vi "Camera Configure.vi"(8 "error in":errorcluster) -> (0 "error out":errorcluster)   [LabVIEW 2012]
doc: "The Grab and Attributes Setup example VI allows the user to view the current attributes and settings, update attribute settings, acquire images continuously, and display the images in an image control."
uses:
  <vilib>/userdefined/High Color/IMAQdx.ctl
  Process Controller 3.0/Control code/Camera/Camera source code/Interface Inputs.ctl
  Process Controller 3.0/Control code/Camera/Camera source code/Rotate.ctl
  Process Controller 3.0/Control code/Camera/Camera source code/Image File Type.ctl
  <vilib>/vision/driver/IMAQdx.llb/IMAQdx Acquisition Mode.ctl
  <vilib>/vision/driver/IMAQdx.llb/IMAQdx Buffer Number Mode.ctl
  DAC project/Calibration and Function folders.ctl
  <vilib>/vision/driver/NI_Vision_Acquisition_Software.lvlib
  Process Controller 3.0/Control code/Camera/Camera SubVIs.lvlib
panel:
  out "Global Rectangle":i32[](array[numeric])
  in  "Grab":bool
  in  "Cancel":bool
  in  "OK":bool
  in  "Tab Contro Mainl":T1(tab)
  in  "Attribute Tree":string(tree)
  in  "Camera Name":T2
  in  "Tab Control":T3(tab)
  in  "U32 Value Control":u32(slide) min=480 max=6291456 step=1 scale=5662310.4..6291456.0
  in  "DBL Value Control":dbl(slide) min=0.0 max=3.999 step=1.0 scale=0.0..3.999
  in  "String Value Control":string
  in  "Enum Value Control":u32(ring) items=["160x120 MJPG 30.00fps", "160x120 YUY2 30.00fps", "176x144 MJPG 30.00fps", "176x144 YUY2 30.00fps", "320x240 MJPG 30.00fps", "320x240 YUY2 30.00fps", "352x288 MJPG 30.00fps", "352x288 YUY2 30.00fps", "640x480 MJPG 30.00fps", "640x480 YUY2 30.00fps", "1024x768 MJPG 30.00fps", "1024x768 YUY2 12.00fps", "1280x720 MJPG 15.00fps", "1280x720 YUY2 10.00fps", "1280x1024 MJPG 15.00fps", "1280x1024 YUY2 7.50fps", "1600x1200 MJPG 15.00fps", "1600x1200 YUY2 5.00fps", "1920x1080 MJPG 15.00fps", "1920x1080 YUY2 4.00fps", "2048x1536 MJPG 15.00fps", "2048x1536 YUY2 3.00fps"]
  in  "Boolean Value Control":bool=TRUE
  in  "Command Value Control":bool
  out "Units":string
  out "Tooltip":string
  out "Image":T4(plugin-control)
  in  "Interface inputs":T5={"Elevation of top of Field of View (cm)"=10.0, "Field of View Height (cm)"=-0.1, "Smooth Length (cm)"=5.0, "Min derivative magnitude"=5.0, "Color Plane"=enum."Green"} {"Smooth Length (cm)" min=0.01 max=1000.0 step=0.1; "Field of View Height (cm)" min=0.1 max=1000.0 step=0.1}
  in  "File Type":T6
  in  "Image Save Rate (s)":dbl=5.0 min=0.05 step=0.05 format="%#_3f"
  in  "Image folder":path
  in  "Record images":bool
  in  "Rotate Image":T7
  out "Buffer Number":u32
  out "Interface elevation":dbl format="%#_3g"
  out "derivative magnitude":dbl format="%#_3g"
  out "Tab Control Ref":T8
  # "These settings are saved in the  ProCoDA configuration file. The Region of Interest is also saved in the configuration file."
  # "Turn of the camera external code in Process Controller prior to using this software. Only one application can interface with the camera at a time. After the camera is configured you can close this application and open the camera external code in Process Controller.\n\nConfigure the camera (light settings, resolution etc.) and then test those settings by acquiring images. \n \nUse the rectangle tool in the image to define the region of interest where the floc water interface will appear.\nThe region of interest is saved in a configuration file.\n\nChoose a folder to save images during the experiment.\nChoose the rate at which images are saved.\n\nUse TIFF files if you plan to do pixel by pixel image analysis and thus don't want image compression. Otherwise JPEG is a good option to reduce file size. \n\nWhen testing to see if the interface is correctly identified, a horizontal black line with a height equal to the smoothing length will appear on the image when an interface is found. If an interface is found, but the line does not appear that is due to the fact the image is reduced in size and the pixels containing the line are not being displayed. You can zoom on the image to see the line."
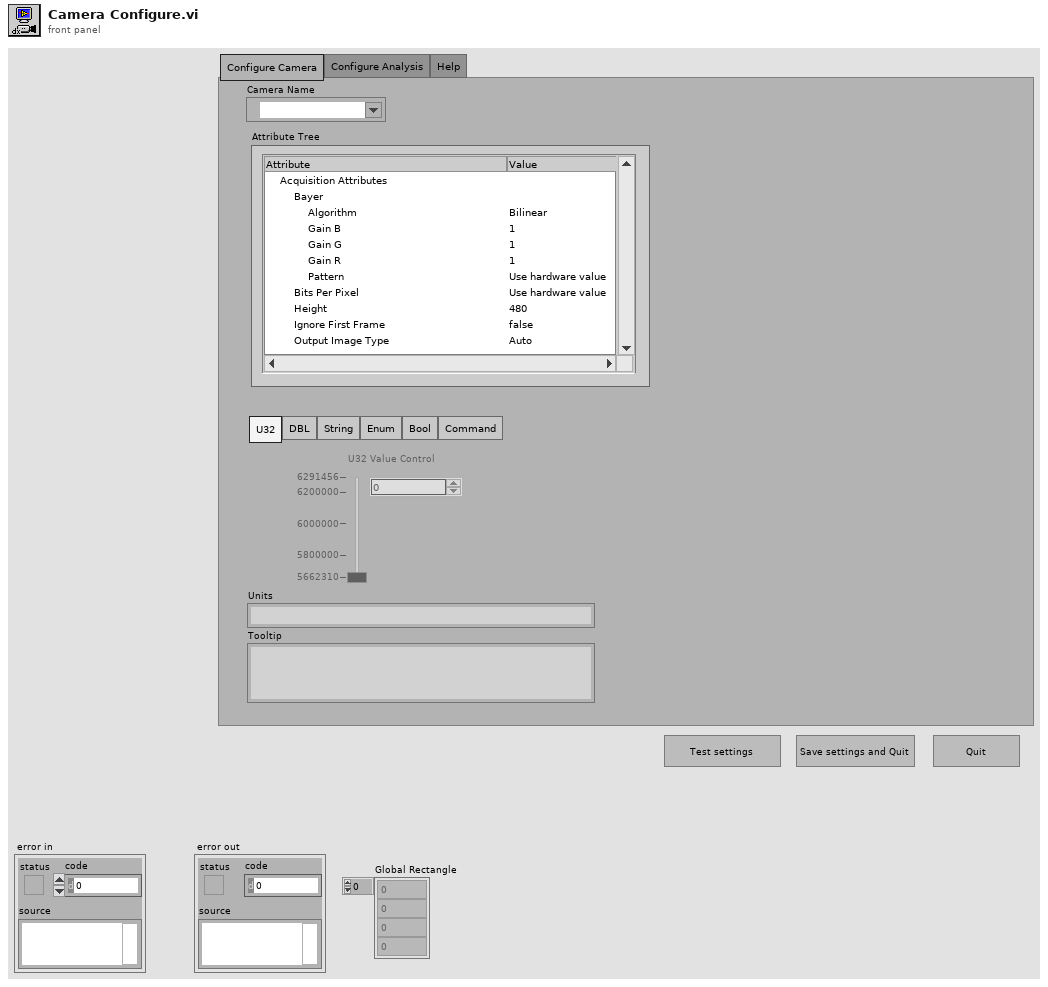
[diagram p1: front panel]
types:
  T1 = enum32{"Configure Camera", "Configure Analysis", "Help"}
  T2 = typedef "IMAQdx.ctl" = refnum<k21>
  T3 = enum32{"U32", "DBL", "String", "Enum", "Bool", "Command"}
  T4 = typedef "IMAQ Image.ctl" = refnum<image>
  T5 = typedef "Camera SubVIs.lvlib/Interface Inputs.ctl" = cluster{"Elevation of top of Field of View (cm)":dbl, "Field of View Height (cm)":dbl, "Smooth Length (cm)":dbl, "Min derivative magnitude":dbl, "Color Plane":enum16{"Red", "Green", "Blue", "Combined"}}
  T6 = typedef "Camera SubVIs.lvlib/Image File Type.ctl" = enum16{"BMP", "JPEG", "JPEG 2000", "PNG", "PNG with Vision Info", "TIFF"}
  T7 = typedef "Camera SubVIs.lvlib/Rotate.ctl" = enum16{"None", "CW", "CCW"}
  T8 = cluster{"Tab Control":refnum<vi>, "U32 Value Control":refnum<vi>, "DBL Value Control":refnum<vi>, "String Value Control":refnum<vi>, "Enum Value Control":refnum<vi>, "Boolean Value Control":refnum<vi>, "Command Value Control":refnum<vi>}
  T9 = enum32{"invalid app kind", "Development System", "Run Time System", "Student Edition", "Embedded LabVIEW", "Evaluation", "Custom"}
  T10 = cluster{"Global Rectangle":i32[], "Contours":cluster{"Contour Type":u32, "ROI Type":u32, "Points":i32[]}[]}
  T11 = typedef "NI_Vision_Acquisition_Software.lvlib/IMAQdx Acquisition Mode.ctl" = enum32{"One Shot", "Continuous"}
  T12 = enum8{"Enabled", "Disabled", "Disabled and Grayed Out"}
  T13 = typedef "Calibration and Function folders.ctl" = enum16{"Sensors", "Functions", "Config File", "UserAppFolder"}
  T14 = typedef "Image Type" = u32
  T15 = typedef "NI_Vision_Acquisition_Software.lvlib/IMAQdx Buffer Number Mode.ctl" = enum32{"Next", "Last", "Buffer Number"}
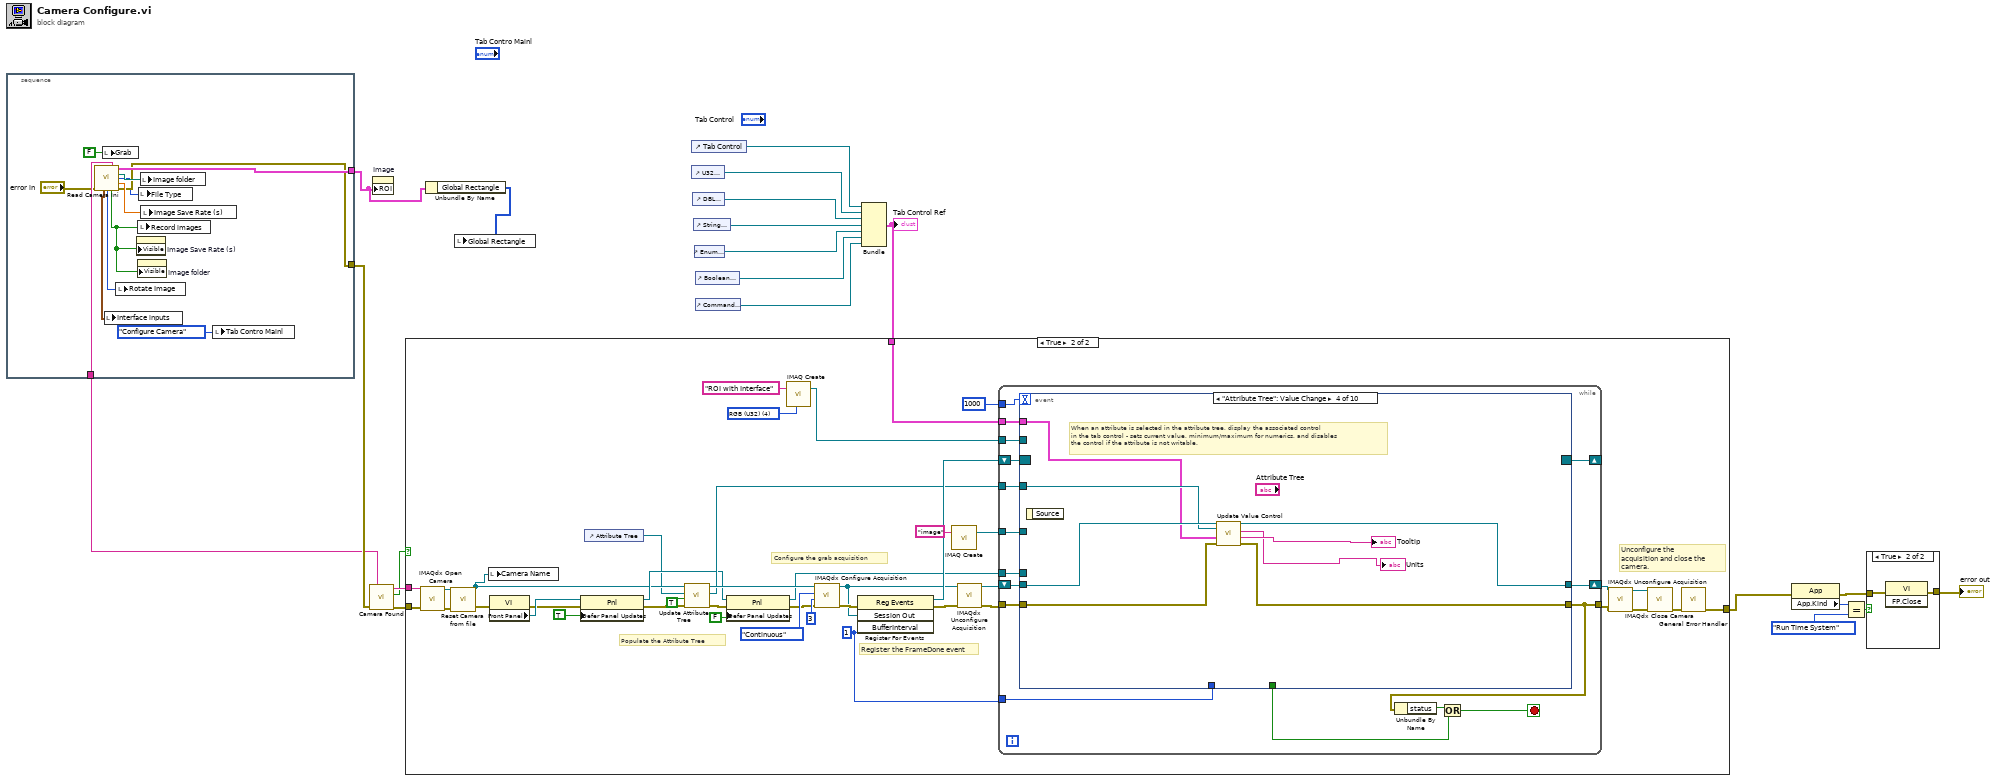
[diagram p0: block diagram]
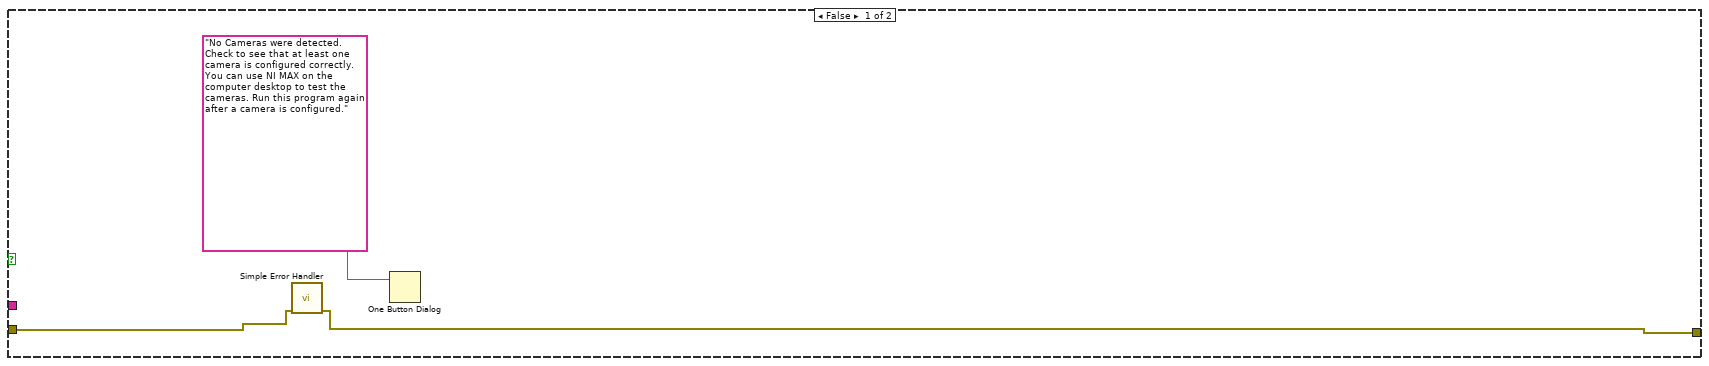
[diagram p3: hidden frame]
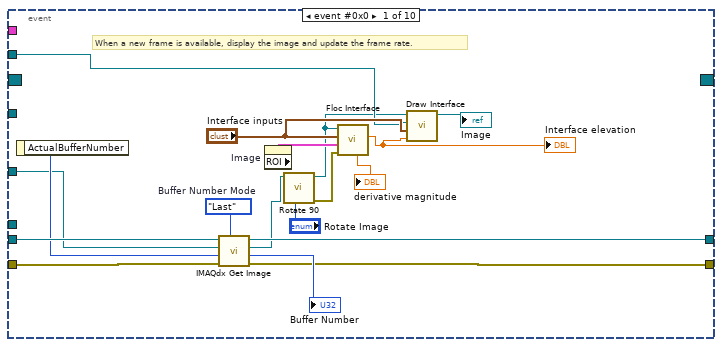
[diagram p4: hidden frame]
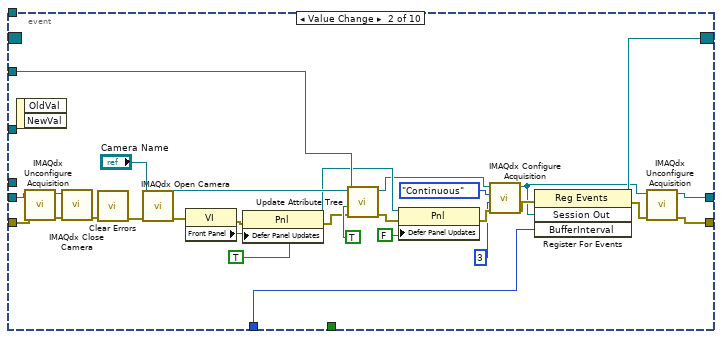
[diagram p5: hidden frame]
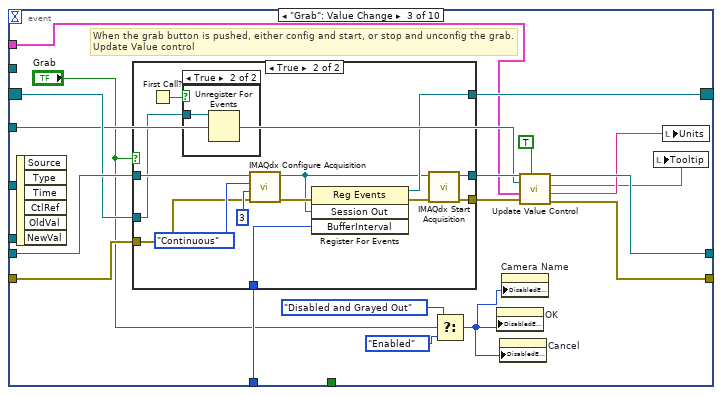
[diagram p6: hidden frame]
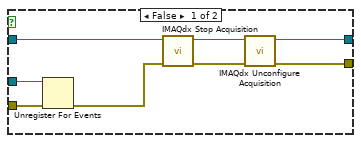
[diagram p7: hidden frame]
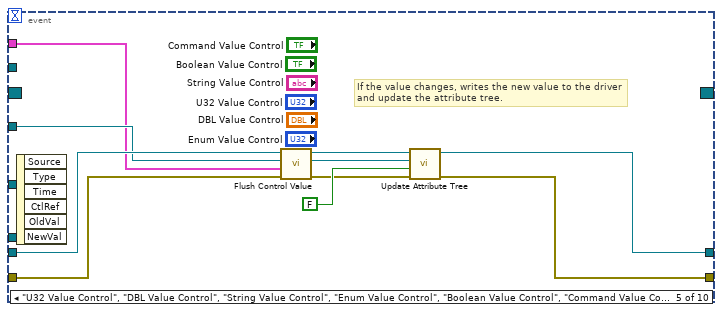
[diagram p9: hidden frame]
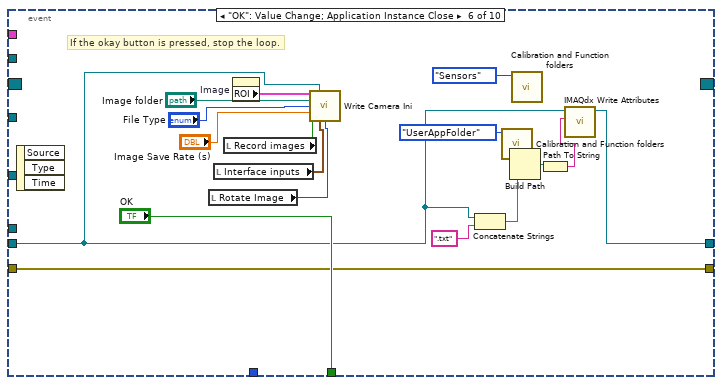
[diagram p10: hidden frame]
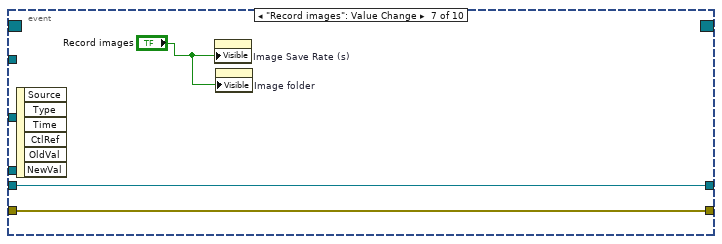
[diagram p11: hidden frame]
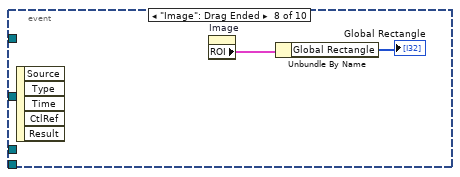
[diagram p12: hidden frame]
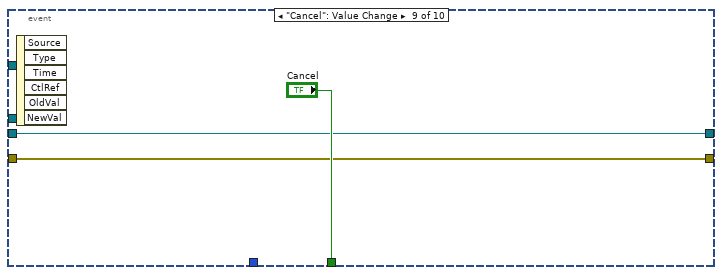
[diagram p13: hidden frame]
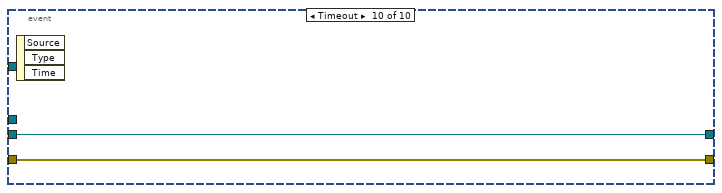
[diagram p14: hidden frame]
diagram:
  n1 = stacked-sequence {
    tunnel: [w33] -> w14
    tunnel: [w24] -> w12
    tunnel: [w26] -> w11
    frame #0 {
      n2 = call "Read Camera Ini.vi"("error in (no error)"="error in") -> ("CameraName"=w26:string, "ROI"=w33:T10, "Image folder"=w31:path, "File Type"=w22:T6, "Image Save Rate (s)"=w30:dbl, "Interface inputs"=w27:T5, "Rotate"=w23:T7, "Record images"=w29:bool, "error out"=w24:errorcluster)  [unwired: 6 in]
      n3 = local write "Grab"(FALSE ("Grab")) -> ()
      n4 = local write "Interface inputs"(w27) -> ()
      n5 = local write "Rotate Image"(w23) -> ()
      n6 = property on="Image Save Rate (s)" class="DigNum (strict)"("Visible"=w29) -> ()  [unwired: 2 in, 2 out]
      n7 = local write "Record images"(w29) -> ()
      n8 = property on="Image folder" class="Path"("Visible"=w29) -> ()  [unwired: 2 in, 2 out]
      n9 = local write "File Type"(w22) -> ()
      n10 = local write "Image folder"(w31) -> ()
      n11 = local write "Image Save Rate (s)"(w30) -> ()
      n12 = local write "Tab Contro Mainl"(T1."Configure Camera" ("Tab Contro Mainl")) -> ()
    }
  }
  n13 = call "Camera Found.vi"("error in"=w12, "CameraName"=w11) -> ("error out"=w9:errorcluster, "Camera Found"=w8:bool, "CameraName out"=w10:string)  [unwired: 7 in]
  n14 = property on="Image" class="ImageControl"("ROI"=w14) -> ()  [unwired: 2 in, 2 out]
  n15 = Unbundle By Name(w14) -> ("Global Rectangle"=w13:i32[])
  n16 = local write "Global Rectangle"(w13) -> ()
  n17 = control-ref of="Tab Control"() -> (w21:refnum<vi>)
  n18 = control-ref of="U32 Value Control"() -> (w19:refnum<vi>)
  n19 = control-ref of="DBL Value Control"() -> (w18:refnum<vi>)
  n20 = control-ref of="String Value Control"() -> (w20:refnum<vi>)
  n21 = control-ref of="Enum Value Control"() -> (w17:refnum<vi>)
  n22 = control-ref of="Boolean Value Control"() -> (w16:refnum<vi>)
  n23 = control-ref of="Command Value Control"() -> (w15:refnum<vi>)
  n24 = Bundle("Tab Control"=w21, "U32 Value Control"=w19, "DBL Value Control"=w18, "String Value Control"=w20, "Enum Value Control"=w17, "Boolean Value Control"=w16, "Command Value Control"=w15) -> (w1:T8)  [unwired: 1 out]
  "Tab Control Ref" <- w1
  n25 = case shown="True" w8 {
    tunnel: [w34 w54] -> w3
    tunnel: w10 -> [_ w44]
    tunnel: w9 -> [w36 w43]
    tunnel: w1 -> [_ w38]
    frame False {
      n26 = call <vilib>:"Simple Error Handler.vi"("error in (no error)"=w36) -> ("error out"=w34:errorcluster)  [unwired: 4 in, 4 out]
      n27 = One Button Dialog(message="No Cameras were detected. Check to see that at least one camera is configured correctly. You can use NI MAX on the computer desktop to test the cameras. Run this program again after a camera is configured.") -> ()  [unwired: 1 in, 1 out]
    }
    frame True {
      w50 = T14 4 items=["Grayscale (U8)", "Grayscale (I16)", "Grayscale (SGL)", "Complex (CSG)", "RGB (U32)", "HSL (U32)", "RGB (U64)", "Grayscale (U16)"] ("Image Type")
      w60 = u32 1 ("BufferInterval")
      # "Unconfigure the acquisition and close the camera."
      # "Register the FrameDone event"
      # "Configure the grab acquisition"
      # "Populate the Attribute Tree"
      n28 = call <vilib>:"IMAQdx Open Camera.vi"("error in"=w43, "Session In"=w44) -> ("error out"=w48:errorcluster, "Session Out"=w47:T2)  [unwired: 1 in, 7 out]
      n29 = call "Reset Camera from file.vi"("error in"=w48, "Refnum in"=w47) -> ("error out"=w46:errorcluster, "Refnum out"=w42:T2)  [unwired: 8 in]
      n30 = local write "Camera Name"(w42) -> ()
      n31 = property class="VI"(error in=w46) -> (error out=w61:errorcluster, "Front Panel"=w62:refnum<vi>)  [unwired: 1 in, 1 out]
      n32 = property class="Pnl"(reference=w62, error in=w61, "Defer Panel Updates"=TRUE) -> (reference out=w65:refnum<vi>, error out=w69:errorcluster)
      n33 = control-ref of="Attribute Tree"() -> (w37:refnum<vi>)
      n34 = call "Update Attribute Tree.vi"("error in"=w69, "Flush Tree?"=TRUE, "Tree Control In"=w37, "Camera Name In"=w42) -> ("error out"=w68:errorcluster, "Tree Control Out"=w70:refnum<vi>, "Session Out"=w72:T2)  [unwired: 5 in]
      n35 = property class="Pnl"(reference=w65, error in=w68, "Defer Panel Updates"=FALSE) -> (reference out=w64:refnum<vi>, error out=w66:errorcluster)
      n36 = call "IMAQ Create"("Image Name"="ROI with Interface", "Image Type"=w50) -> ("New Image"=w49:T4)  [unwired: 3 in, 1 out]
      n37 = call <vilib>:"IMAQdx Configure Acquisition.vi"("error in"=w66, "Number of Buffers"=u32 3, "Continuous?"=IMAQdx_Acquisition_Mode."Continuous", "Session In"=w72) -> ("error out"=w75:errorcluster, "Session Out"=w57:T2)  [unwired: 6 out]
      n38 = register-events(error in=w75, w57, w60) -> (reference out=w74:refnum<event-registration>, error out=w59:errorcluster)  [unwired: 1 in]
      n39 = call "IMAQ Create"("Image Name"="image") -> ("New Image"=w52:T4)  [unwired: 3 in, 2 out]
      n40 = call <vilib>:"IMAQdx Unconfigure Acquisition.vi"("error in"=w59, "Session In"=w57) -> ("error out"=w58:errorcluster, "Session Out"=w56:T2)  [unwired: 8 out]
      n41 = while {
        tunnel: w58 -> [w90]
        tunnel: [w88] -> w55
        tunnel: w52 -> [w89]
        tunnel: 1000 -> [w86]
        tunnel: w70 -> [w85]
        tunnel: w64 -> [w84]
        tunnel: w60 -> [w82]
        shift-right: [w81] -> _
        shift-left: w74 -> [w87]
        shift-right: [w80] -> w53
        shift-left: w56 -> [w91]
        tunnel: w49 -> [w79]
        tunnel: w38 -> [w78]
        stop <- w93 stop-if-true
        n42 = event shown="[3] \"Attribute Tree\": Value Change" {
          selector: w87 -> [_ _ w155 _ _ _ _ _ _ _]
          dyn-events: [_ w118 w157 _ _ _ _ _ _ _] -> w81
          timeout: w86 -> [_ _ _ _ _ _ _ _ _ _]
          tunnel: w91 -> [w111 w139 w158 w188 w197 w205 w218 _ w223 w225]
          tunnel: w90 -> [w110 w138 w154 w186 w198 w215 w217 _ w222 w226]
          tunnel: w89 -> [w103 _ _ _ _ _ _ _ _ _]
          tunnel: [w104 w114 w152 w187 w192 w210 w218 _ w223 w225] -> w80
          tunnel: [w99 w116 w150 w185 w189 w215 w217 _ w222 w226] -> w88
          tunnel: w85 -> [_ w136 w149 w184 w195 _ _ _ _ _]
          tunnel: w84 -> [_ _ _ _ _ _ _ _ _ _]
          tunnel: [_ _ _ _ _ "OK" _ _ "Cancel" _] -> w83
          tunnel: w82 -> [_ w119 w156 _ _ _ _ _ _ _]
          tunnel: w79 -> [w100 _ _ _ _ _ _ _ _ _]
          tunnel: w78 -> [_ _ w141 w183 w191 _ _ _ _ _]
          event event #0x0 {
            w109 = IMAQdx_Buffer_Number_Mode."Last"  # Buffer Number Mode
            # "When a new frame is available, display the image and update the frame rate."
            n43 = event-data() -> ("ActualBufferNumber"=w108:u32)  [unwired: 1 out]
            n44 = call <vilib>:"IMAQdx Get Image.vi"("Buffer Number Mode (Next)"=w109, "error in"=w110, "Buffer Number In"=w108, "Image In"=w103, "Session In"=w111) -> ("error out"=w99:errorcluster, "Buffer Number Out"=→"Buffer Number":u32, "Image Out"=w97:T4, "Session Out"=w104:T2)  [unwired: 3 out]
            n45 = property on="Image" class="ImageControl"() -> ("ROI"=w106:T10)  [unwired: 2 in, 2 out]
            n46 = call "Rotate 90.vi"("Rotate"="Rotate Image", "Image Src"=w97) -> ("error out"=w94:errorcluster, "Image Dst Out"=w96:T4)  [unwired: 8 in]
            n47 = call "Floc Interface.vi"("error in"=w94, "ROI"=w106, "Interface inputs"="Interface inputs", "Image"=w96) -> ("Interface elevation"=w102:dbl, "min value"=→"derivative magnitude":dbl)  [unwired: 4 in, 2 out]
            "Interface elevation" <- w102
            n48 = call "Draw Interface.vi"("Interface elevation"=w102, "Interface inputs"="Interface inputs", "Image Dst"=w100, "Image"=w96) -> ("Image out"=→"Image":T4)  [unwired: 7 in]
          }
          event Value Change {
            n49 = event-data() -> ()  [unwired: 3 out]
            n50 = call <vilib>:"IMAQdx Unconfigure Acquisition.vi"("error in"=w138, "Session In"=w139) -> ("error out"=w140:errorcluster, "Session Out"=w137:T2)  [unwired: 8 out]
            n51 = call <vilib>:"IMAQdx Close Camera.vi"("error in"=w140, "Session In"=w137) -> ("error out"=w133:errorcluster)  [unwired: 9 out]
            n52 = call <vilib>:"Clear Errors.vi"("error in (no error)"=w133) -> ("error out"=w132:errorcluster)  [unwired: 6 in]
            n53 = call <vilib>:"IMAQdx Open Camera.vi"("error in"=w132, "Session In"="Camera Name") -> ("error out"=w129:errorcluster, "Session Out"=w134:T2)  [unwired: 1 in, 7 out]
            n54 = property class="VI"(error in=w129) -> (error out=w131:errorcluster, "Front Panel"=w113:refnum<vi>)  [unwired: 1 in, 1 out]
            n55 = property class="Pnl"(reference=w113, error in=w131, "Defer Panel Updates"=TRUE) -> (reference out=w125:refnum<vi>, error out=w128:errorcluster)
            n56 = call "Update Attribute Tree.vi"("error in"=w128, "Flush Tree?"=TRUE, "Tree Control In"=w136, "Camera Name In"=w134) -> ("error out"=w126:errorcluster, "Session Out"=w121:T2)  [unwired: 5 in, 1 out]
            n57 = property class="Pnl"(reference=w125, error in=w126, "Defer Panel Updates"=FALSE) -> (error out=w124:errorcluster)  [unwired: 1 out]
            n58 = call <vilib>:"IMAQdx Configure Acquisition.vi"("error in"=w124, "Number of Buffers"=u32 3, "Continuous?"=IMAQdx_Acquisition_Mode."Continuous", "Session In"=w121) -> ("error out"=w120:errorcluster, "Session Out"=w115:T2)  [unwired: 6 out]
            n59 = register-events(error in=w120, w115, w119) -> (reference out=w118:refnum<event-registration>, error out=w117:errorcluster)  [unwired: 1 in]
            n60 = call <vilib>:"IMAQdx Unconfigure Acquisition.vi"("error in"=w117, "Session In"=w115) -> ("error out"=w116:errorcluster, "Session Out"=w114:T2)  [unwired: 8 out]
          }
          event "Grab": Value Change {
            # "When the grab button is pushed, either config and start, or stop and unconfig the grab.\nUpdate Value control"
            n61 = event-data() -> ()  [unwired: 7 out]
            n62 = case shown="True" "Grab" {
              tunnel: w158 -> [w166 w177]
              tunnel: [w163 w179] -> w153
              tunnel: [w162 w178] -> w151
              tunnel: [_ w172] -> w157
              tunnel: w156 -> [_ w170]
              tunnel: w155 -> [w161 w168]
              tunnel: w154 -> [w159 w169]
              frame False {
                n63 = Unregister For Events(event registration refnum=w161, error in=w159) -> (error out=w160:errorcluster)
                n64 = call <vilib>:"IMAQdx Stop Acquisition.vi"("error in"=w160, "Session In"=w166) -> ("error out"=w164:errorcluster, "Session Out"=w165:T2)  [unwired: 8 out]
                n65 = call <vilib>:"IMAQdx Unconfigure Acquisition.vi"("error in"=w164, "Session In"=w165) -> ("error out"=w162:errorcluster, "Session Out"=w163:T2)  [unwired: 8 out]
              }
              frame True {
                n66 = First Call?() -> (First Call?: T/F=w167:bool)
                n67 = case shown="True" w167 {
                  tunnel: w168 -> [_ w180]
                  frame False {
                  }
                  frame True {
                    n68 = Unregister For Events(event registration refnum=w180) -> ()  [unwired: 1 in, 1 out]
                  }
                }
                n69 = call <vilib>:"IMAQdx Configure Acquisition.vi"("error in"=w169, "Number of Buffers"=u32 3, "Continuous?"=IMAQdx_Acquisition_Mode."Continuous", "Session In"=w177) -> ("error out"=w174:errorcluster, "Session Out"=w171:T2)  [unwired: 6 out]
                n70 = register-events(error in=w174, w171, w170) -> (reference out=w172:refnum<event-registration>, error out=w173:errorcluster)  [unwired: 1 in]
                n71 = call <vilib>:"IMAQdx Start Acquisition.vi"("error in"=w173, "Session In"=w171) -> ("error out"=w178:errorcluster, "Session Out"=w179:T2)  [unwired: 8 out]
              }
            }
            n72 = Select(t=T12."Disabled and Grayed Out" ("Disabled"), s="Grab", f=T12."Enabled" ("Disabled")) -> (s? t:f=w142:T12)
            n73 = property on="OK" class="Bool"("DisabledEnum"=w142) -> ()  [unwired: 2 in, 2 out]
            n74 = property on="Cancel" class="Bool"("DisabledEnum"=w142) -> ()  [unwired: 2 in, 2 out]
            n75 = property on="Camera Name" class="IMAQdx (strict)"("DisabledEnum"=w142) -> ()  [unwired: 2 in, 2 out]
            n76 = call "Update Value Control.vi"("Force update?"=TRUE, "error in (no error)"=w151, "Tab Control Ref In"=w141, "Tree Control In"=w149, "Session In"=w153) -> ("error out"=w150:errorcluster, "Units"=w148:string, "Tooltip"=w147:string, "Session Out"=w152:T2)  [unwired: 3 in]
            n77 = local write "Tooltip"(w147) -> ()
            n78 = local write "Units"(w148) -> ()
          }
          event "Attribute Tree": Value Change {
            # "When an attribute is selected in the attribute tree, display the associated control\nin the tab control - sets current value, minimum/maximum for numerics, and disables\nthe control if the attribute is not writable."
            n79 = event-data() -> ()  [unwired: 2 out]
            n80 = call "Update Value Control.vi"("error in (no error)"=w186, "Tab Control Ref In"=w183, "Tree Control In"=w184, "Session In"=w188) -> ("error out"=w185:errorcluster, "Units"=→"Tooltip":string, "Tooltip"=→"Units":string, "Session Out"=w187:T2)  [unwired: 4 in]
          }
          event "U32 Value Control", "DBL Value Control", "String Value Control", "Enum Value Control", "Boolean Value Control", "Command Value Control": Value Change {
            # "If the value changes, writes the new value to the driver\nand update the attribute tree."
            n81 = event-data() -> ()  [unwired: 7 out]
            n82 = call "Flush Control Value.vi"("error in (no error)"=w198, "Tab Control Ref In"=w191, "Tree Control In"=w195, "Session In"=w197) -> ("error out"=w190:errorcluster, "Tree Control Out"=w194:refnum<vi>, "Session Out"=w196:T2)  [unwired: 5 in]
            n83 = call "Update Attribute Tree.vi"("error in"=w190, "Flush Tree?"=FALSE, "Tree Control In"=w194, "Camera Name In"=w196) -> ("error out"=w189:errorcluster, "Session Out"=w192:T2)  [unwired: 5 in, 1 out]
          }
          event "OK": Value Change; Application Instance Close {
            # "If the okay button is pressed, stop the loop."
            n84 = event-data() -> ()  [unwired: 4 out]
            n85 = local read "Rotate Image"() -> (w199:T7)
            n86 = local read "Interface inputs"() -> (w207:T5)
            n87 = local read "Record images"() -> (w208:bool)
            n88 = property on="Image" class="ImageControl"() -> ("ROI"=w214:T10)  [unwired: 2 in, 2 out]
            n89 = call "Write Camera Ini.vi"("ROI"=w214, "CameraName"=w205, "Image folder"="Image folder", "File Type"="File Type", "Image Save Rate (s)"="Image Save Rate (s)", "Record images"=w208, "Interface inputs"=w207, "Rotate"=w199) -> ()  [unwired: 8 in]
            n90 = Concatenate Strings(w205, ".txt") -> (w204:string)
            n91 = call "Calibration and Function folders.vi"("Folder"=Calibration_and_Function_folders."UserAppFolder") -> ("Selected Folder"=w201:path)  [unwired: 10 in]
            n92 = Build Path(base path=w201, name or relative path=w204) -> (appended path=w211:path)
            n93 = call "Calibration and Function folders.vi"("Folder"=Calibration_and_Function_folders."Sensors") -> ()  [unwired: 10 in, 1 out]
            n94 = Path To String(path=w211) -> (string=w209:string)
            n95 = call <vilib>:"IMAQdx Write Attributes.vi"("Filename"=w209, "Session In"=w205) -> ("Session Out"=w210:T2)  [unwired: 8 in, 1 out]
          }
          event "Record images": Value Change {
            n96 = event-data() -> ()  [unwired: 7 out]
            n97 = property on="Image Save Rate (s)" class="DigNum (strict)"("Visible"="Record images") -> ()  [unwired: 2 in, 2 out]
            n98 = property on="Image folder" class="Path"("Visible"="Record images") -> ()  [unwired: 2 in, 2 out]
          }
          event "Image": Drag Ended {
            n99 = event-data() -> ()  [unwired: 6 out]
            n100 = property on="Image" class="ImageControl"() -> ("ROI"=w221:T10)  [unwired: 2 in, 2 out]
            n101 = Unbundle By Name(w221) -> ("Global Rectangle"=→"Global Rectangle":i32[])
          }
          event "Cancel": Value Change {
            n102 = event-data() -> ()  [unwired: 7 out]
          }
          event Timeout {
            n103 = event-data() -> ()  [unwired: 4 out]
          }
        }
        n104 = Unbundle By Name(w88) -> ("status"=w92:bool)
        n105 = Or(x=w92, y=w83) -> (x .or. y?=w93:bool)
      }
      n106 = call <vilib>:"IMAQdx Unconfigure Acquisition.vi"("error in"=w55, "Session In"=w53) -> ("error out"=w41:errorcluster, "Session Out"=w40:T2)  [unwired: 8 out]
      n107 = call <vilib>:"IMAQdx Close Camera.vi"("error in"=w41, "Session In"=w40) -> ("error out"=w39:errorcluster)  [unwired: 9 out]
      n108 = call <vilib>:"General Error Handler.vi"("error in (no error)"=w39) -> ("error out"=w54:errorcluster)  [unwired: 1 in, 13 out]
    }
  }
  n109 = property class="App"(error in=w3) -> (error out=w7:errorcluster, "App.Kind"=w5:T9)  [unwired: 1 in, 1 out]
  n110 = Equal?(x=w5, y=T9."Run Time System" ("Application:Kind")) -> (x = y?=w6:bool)
  n111 = case shown="True" w6 {
    tunnel: w7 -> [w227 w229]
    tunnel: [w227 w228] -> w4
    frame False {
    }
    frame True {
      n112 = invoke class="VI" method="FP.Close"(error in=w229) -> (error out=w228:errorcluster)  [unwired: 2 in, 2 out]
    }
  }
  "error out" <- w4
